vi "provision shop.vi"() -> ()   [LabVIEW 2017]
panel:
  out "result 2":i16
  in  "quantity 9":u8
  in  "item1 9":bool
  in  "quantity 8":u8
  in  "item1 8":bool
  in  "quantity 7":u8
  in  "item1 7":bool
  in  "quantity 6":u8
  in  "item1 6":bool
  in  "item1":bool
  in  "quantity":u8=1 min=1 max=10
  # "provision bill"
  # "10"
  # "20"
  # "20"
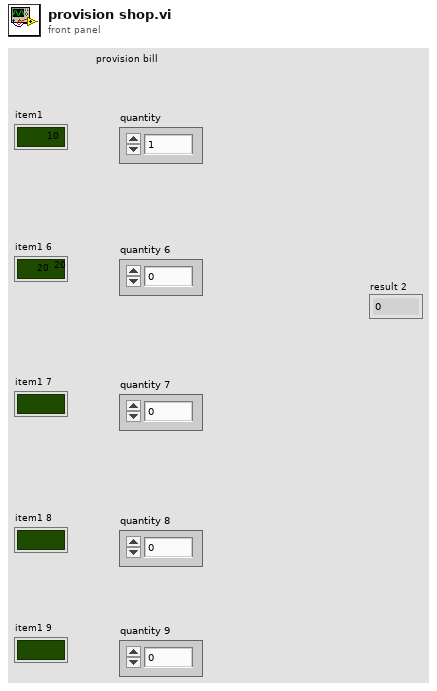
[diagram p1: front panel]
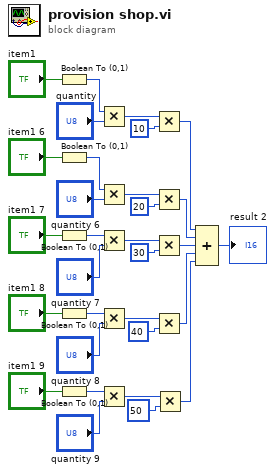
[diagram p0: block diagram]
diagram:
  n1 = Boolean To (0,1)(Boolean="item1") -> (0, 1=w31:i16)
  n2 = Boolean To (0,1)(Boolean="item1 6") -> (0, 1=w22:i16)
  n3 = Boolean To (0,1)(Boolean="item1 7") -> (0, 1=w21:i16)
  n4 = Boolean To (0,1)(Boolean="item1 8") -> (0, 1=w13:i16)
  n5 = Boolean To (0,1)(Boolean="item1 9") -> (0, 1=w12:i16)
  n6 = Multiply(x=w31, y="quantity") -> (x*y=w29:i16)
  n7 = Multiply(x=w22, y="quantity 6") -> (x*y=w24:i16)
  n8 = Multiply(x=w21, y="quantity 7") -> (x*y=w1:i16)
  n9 = Multiply(x=w13, y="quantity 8") -> (x*y=w15:i16)
  n10 = Multiply(x=w12, y="quantity 9") -> (x*y=w10:i16)
  n11 = Multiply(x=w29, y=i16 10) -> (x*y=w7:i16)
  n12 = Multiply(x=w24, y=i16 20) -> (x*y=w6:i16)
  n13 = Multiply(x=w1, y=i16 30) -> (x*y=w5:i16)
  n14 = Multiply(x=w15, y=i16 40) -> (x*y=w4:i16)
  n15 = Multiply(x=w10, y=i16 50) -> (x*y=w3:i16)
  n16 = Compound Arithmetic op=ADD(w7, w6, w5, w4, w3) -> (→"result 2":i16)
